vi "Waveform Scan Done.vi"(8 "error in (no error)":errorcluster, 11 "Model in":refnum<class "Model.lvclass">) -> (0 "error out":errorcluster, 2 "Done":bool, 3 "Model out":refnum<class "Model.lvclass">)   [LabVIEW 2016]
uses:
  Model.lvclass
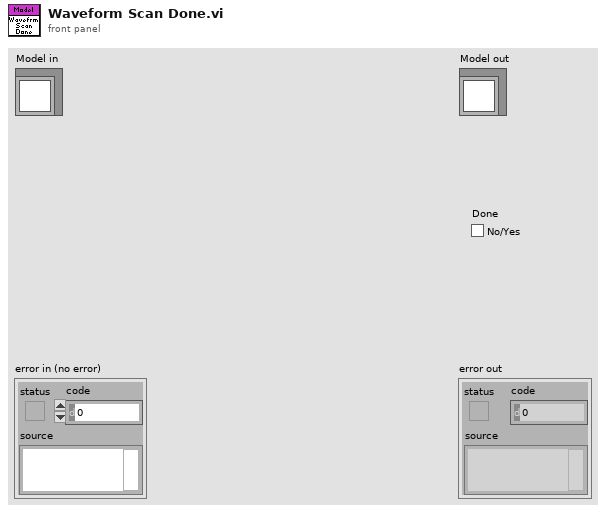
[diagram p1: front panel]
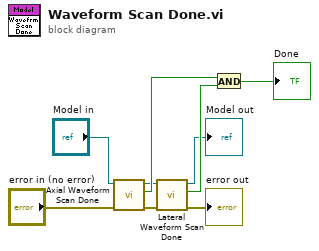
[diagram p0: block diagram]
diagram:
  n1 = call "Axial Waveform Scan Done.vi"("error in (no error)"="error in (no error)", "Model in"="Model in") -> ("error out"=w2:errorcluster, "Done"=w8:bool, "Model out"=w1:refnum<class "Model.lvclass">)  [unwired: 7 in]
  n2 = call "Lateral Waveform Scan Done.vi"("error in (no error)"=w2, "Model in"=w1) -> ("error out"=→"error out":errorcluster, "Done"=w9:bool, "Model out"=→"Model out":refnum<class "Model.lvclass">)  [unwired: 7 in]
  n3 = And(x=w8, y=w9) -> (x .and. y?=→"Done":bool)
